vi "Host Main.vi"() -> ()   [LabVIEW 2015]
doc: "This application launches and executes the Tag Bus Data framework configuration for the specified target alias. This is a simple example of the framework API functions, but may also be a suitable starting point for a Host UI or Thick Client that is running a local version of the framework."
uses:
  <vilib>/NI/Module Execution Interface/Engine Runtime/Execution States.ctl
  <vilib>/NI/Module Execution Interface/Engine Runtime/Fault.ctl
  <vilib>/NI/Tag Bus Module Framework/runtime/error classification.ctl
  <vilib>/NI/Current Value Table/DataTypes/Double_Read.vi
  <vilib>/NI/Current Value Table/DataTypes/U64_Read.vi
  <vilib>/NI/Current Value Table/DataTypes/U32_Read.vi
  <vilib>/NI/Current Value Table/DataTypes/Boolean_Read.vi
  <vilib>/NI/Current Value Table/Type to Enum.vi
  <vilib>/NI/Current Value Table/DataTypes/Double_Type To Enum.vi
  <vilib>/NI/Current Value Table/DataTypes/U64_Type To Enum.vi
  <vilib>/NI/Current Value Table/DataTypes/U32_Type To Enum.vi
  <vilib>/NI/Current Value Table/DataTypes/Boolean_Type To Enum.vi
  <vilib>/NI/Current Value Table/FGVs/CVT Globals.vi
  <vilib>/NI/Current Value Table/FGVs/Tag Memory.vi
  <vilib>/NI/Current Value Table/Memory Block.vi
  <vilib>/NI/Current Value Table/DataTypes/Boolean_Memory Block.vi
  <vilib>/NI/Current Value Table/DataTypes/U32_Memory Block.vi
  <vilib>/NI/Current Value Table/DataTypes/U64_Memory Block.vi
  <vilib>/NI/Current Value Table/DataTypes/Double_Memory Block.vi
  <vilib>/NI/Module Execution Interface/Engine Runtime/Engine Runtime Interface.lvclass
  <vilib>/NI/DCAF/Tag Editor Core/Framework Configuration Classes/target runtime/PL_Target Runtime.lvclass
  <vilib>/NI/Tag Bus Module Framework/runtime/TBM module execution interface.lvclass
  <vilib>/NI/Current Value Table/Current Value Table.lvlib
panel:
  out "Exec Time":u64
  out "Iterate DT":u64
  out "Late Count":u32
  out "Late":bool
  out "error out":errorcluster
  out "Duration Outputs":dbl
  out "Duration Process":dbl
  out "Duration Inputs":dbl
  out "Iter Start Time":dbl
  in  "configuration file path":path=path "C:/Git/Benchmarks/Source/Benchmark_10_increments.pcfg"
  in  "target alias":string="DCAF-9030"
  out "engine status":T4(array[cluster])
  in  "stop":bool
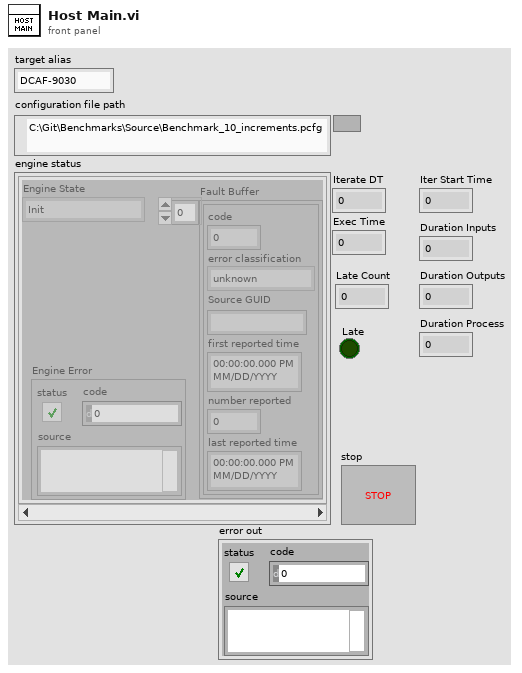
[diagram p1: front panel]
types:
  T1 = typedef "Engine Runtime Interface.lvclass/Execution States.ctl" = enum16{"Init", "Pre-Operational", "Safe-Operational", "Operational", "Stopped"}
  T2 = typedef "Engine Runtime Interface.lvclass/Fault.ctl" = cluster{"code":i32, "error classification":T3, "Source GUID":string, "first reported time":timestamp, "number reported":u32, "last reported time":timestamp}
  T3 = typedef "TBM module execution interface.lvclass/error classification.ctl" = enum16{"unknown", "none", "trivial", "recoverable", "critical"}
  T4 = cluster{"Engine State":T1, "Fault Buffer":T2[], "Engine Error":errorcluster}[]
  T5 = cluster{"Engine State":T1, "Fault Buffer":T2[], "Engine Error":errorcluster}
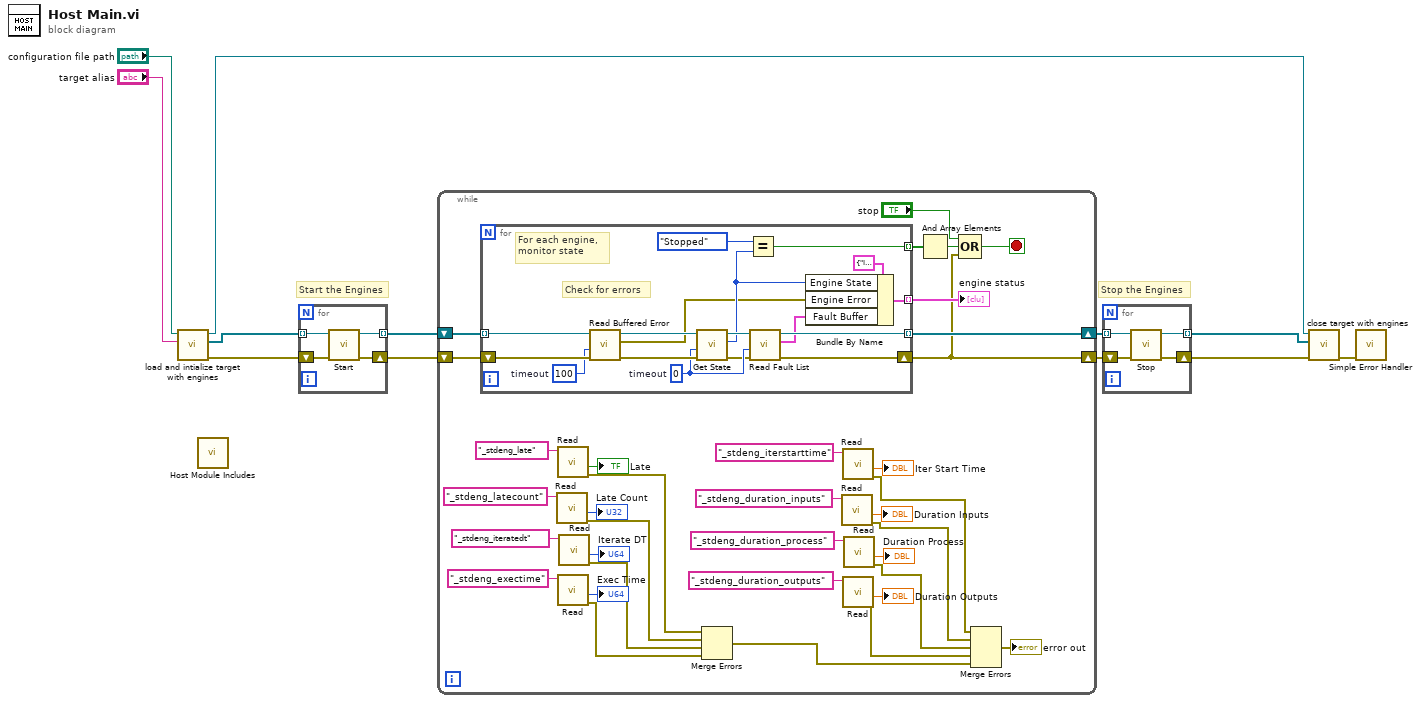
[diagram p0: block diagram]
diagram:
  # "Start the Engines"
  # "Stop the Engines"
  n1 = call <vilib>:"load and intialize target with engines.vi"("target alias"="target alias", "file path"="configuration file path") -> ("error out"=w9:errorcluster, "engine runtime interfaces"=w8:refnum<class "Engine Runtime Interface.lvclass">[], "target runtime"=w5:refnum<class "PL_Target Runtime.lvclass">)  [unwired: 7 in]
  n2 = call "Host Module Includes.vi"() -> ()  [unwired: 12 in]
  n3 = for {
    tunnel: [w16] -> w12 mode=indexing
    tunnel: w8 -> [w13] mode=indexing
    shift-right: [w15] -> w2
    shift-left: w9 -> [w14]
    n4 = call-dynamic "Start.vi"("error in"=w14, "Engine Runtime Interface in"=w13) -> ("error out"=w15:errorcluster, "Engine Runtime Interface out"=w16:refnum<class "Engine Runtime Interface.lvclass">)  [unwired: 8 in]
  }
  n5 = while {
    shift-right: [w49] -> w11
    shift-left: w12 -> [w51]
    shift-right: [w43] -> w10
    shift-left: w2 -> [w50]
    stop <- w47 stop-if-true
    n6 = for {
      tunnel: w51 -> [w68] mode=indexing
      tunnel: [w60] -> w49 mode=indexing
      tunnel: [w63] -> w45 mode=indexing
      shift-right: [w59] -> w43
      shift-left: w50 -> [w67]
      tunnel: [w55] -> w46 mode=indexing
      w58 = 0  # timeout
      w62 = 100  # timeout
      # "For each engine, \nmonitor state"
      # "Check for errors"
      n7 = call-dynamic "Read Buffered Error.vi"("error in"=w67, "timeout in ms (0)"=w62, "Engine Runtime Interface in"=w68) -> ("error out"=w65:errorcluster, "Engine Error"=w53:errorcluster, "Engine Runtime Interface out"=w66:refnum<class "Engine Runtime Interface.lvclass">)  [unwired: 6 in]
      n8 = call-dynamic "Get State.vi"("error in"=w65, "timeout (-1)"=w58, "Engine Runtime Interface in"=w66) -> ("error out"=w52:errorcluster, "Engine State"=w57:T1, "Engine Runtime Interface out"=w61:refnum<class "Engine Runtime Interface.lvclass">)  [unwired: 6 in]
      n9 = Equal?(x=Execution_States."Stopped" ("Engine State"), y=w57) -> (x = y?=w63:bool)
      n10 = call-dynamic "Read Fault List.vi"("error in"=w52, "timeout (-1)"=w58, "Engine Runtime Interface in"=w61) -> ("error out"=w59:errorcluster, "faults"=w56:T2[], "Engine Runtime Interface out"=w60:refnum<class "Engine Runtime Interface.lvclass">)  [unwired: 6 in]
      n11 = Bundle By Name(cluster=T5 {"Engine State"=enum."Init", "Fault Buffer"=[], "Engine Error"={"status"=FALSE, "code"=0, "source"=""}}, "Engine State"=w57, "Engine Error"=w53, "Fault Buffer"=w56) -> (w55:T5)
    }
    "engine status" <- w46
    n12 = call-poly <vilib>:"Read.vi"("Tag Name"="_stdeng_latecount") -> ("error out"=w25:errorcluster, "Value"=→"Late Count":u32)  [unwired: 9 in]
    n13 = call-poly <vilib>:"Read.vi"("Tag Name"="_stdeng_late") -> ("error out"=w26:errorcluster, "Value"=→"Late":bool)  [unwired: 9 in]
    n14 = call-poly <vilib>:"Read.vi"("Tag Name"="_stdeng_exectime") -> ("error out"=w23:errorcluster, "Value"=→"Exec Time":u64)  [unwired: 9 in]
    n15 = call-poly <vilib>:"Read.vi"("Tag Name"="_stdeng_iteratedt") -> ("error out"=w24:errorcluster, "Value"=→"Iterate DT":u64)  [unwired: 9 in]
    n16 = Merge Errors(w26, w25, w24, w23) -> (w22:errorcluster)
    n17 = call-poly <vilib>:"Read.vi"("Tag Name"="_stdeng_duration_inputs") -> ("error out"=w29:errorcluster, "Value"=→"Duration Inputs":dbl)  [unwired: 9 in]
    n18 = call-poly <vilib>:"Read.vi"("Tag Name"="_stdeng_iterstarttime") -> ("error out"=w30:errorcluster, "Value"=→"Iter Start Time":dbl)  [unwired: 9 in]
    n19 = call-poly <vilib>:"Read.vi"("Tag Name"="_stdeng_duration_outputs") -> ("error out"=w27:errorcluster, "Value"=→"Duration Outputs":dbl)  [unwired: 9 in]
    n20 = call-poly <vilib>:"Read.vi"("Tag Name"="_stdeng_duration_process") -> ("error out"=w28:errorcluster, "Value"=→"Duration Process":dbl)  [unwired: 9 in]
    n21 = And Array Elements(Boolean array=w45) -> (logical AND=w44:bool)
    n22 = Compound Arithmetic op=OR("stop", w44, w43) -> (w47:bool)
    n23 = Merge Errors(w30, w29, w28, w27, w22) -> (→"error out":errorcluster)
  }
  n24 = for {
    tunnel: w11 -> [w72] mode=indexing
    shift-right: [w69] -> w4
    shift-left: w10 -> [w71]
    tunnel: [w70] -> w6 mode=indexing
    n25 = call-dynamic "Stop.vi"("error in"=w71, "Engine Runtime Interface in"=w72) -> ("error out"=w69:errorcluster, "Engine Runtime Interface out"=w70:refnum<class "Engine Runtime Interface.lvclass">)  [unwired: 8 in]
  }
  n26 = call <vilib>:"close target with engines.vi"("error in"=w4, "Engine Runtime Interfaces"=w6, "Target Runtime"=w5) -> ("error out"=w1:errorcluster)  [unwired: 8 in]
  n27 = call <vilib>:"Simple Error Handler.vi"("error in (no error)"=w1) -> ()  [unwired: 4 in, 5 out]
